vi "Parse ISO 8601 Timestring.vi"(8 "error in (no error)":errorcluster, 10 "ISO 8601 type":T1, 11 "ISO 8601 Timestring":string) -> (0 "error out":errorcluster, 3 "Time Stamp":timestamp)   [LabVIEW 2013]
uses:
  Controls/ISO 8601 Type.ctl
  Database.lvlib
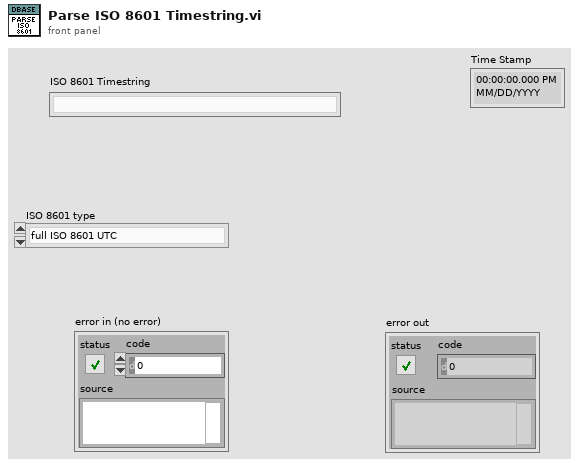
[diagram p1: front panel]
types:
  T1 = typedef "Database.lvlib/ISO 8601 Type.ctl" = enum16{"full ISO 8601 UTC", "Windows ISO 8601 UTC", "YYYY-MM-DD UTC"}
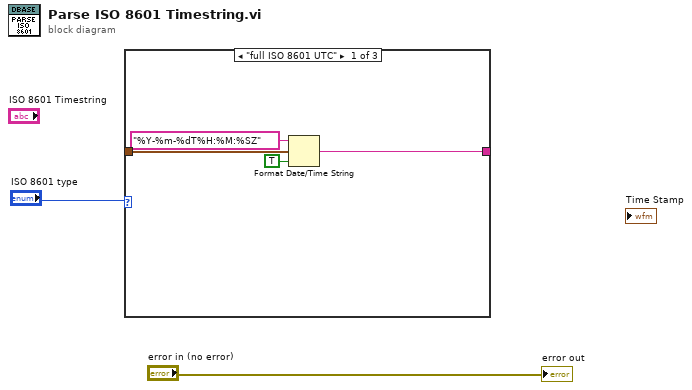
[diagram p0: block diagram]
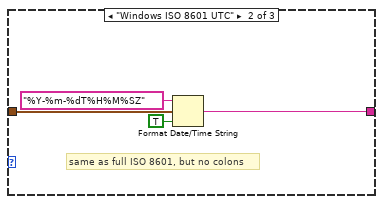
[diagram p2: hidden frame]
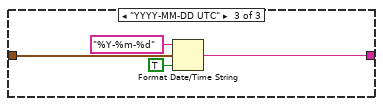
[diagram p3: hidden frame]
diagram:
  n1 = case shown="\"full ISO 8601 UTC\"" "ISO 8601 type" {
    tunnel: [w8 w12 w16] -> w3
    tunnel: [w6 w10 w14] -> w2
    frame "full ISO 8601 UTC" {
      n2 = Format Date/Time String(time format string (%c)="%Y-%m-%dT%H:%M:%SZ", seconds (now)=w8, UTC format=TRUE) -> (date/time string=w6:string)
    }
    frame "Windows ISO 8601 UTC" {
      # "same as full ISO 8601, but no colons"
      n3 = Format Date/Time String(time format string (%c)="%Y-%m-%dT%H%M%SZ", seconds (now)=w12, UTC format=TRUE) -> (date/time string=w10:string)
    }
    frame "YYYY-MM-DD UTC" {
      n4 = Format Date/Time String(time format string (%c)="%Y-%m-%d", seconds (now)=w16, UTC format=TRUE) -> (date/time string=w14:string)
    }
  }
  "error out" <- "error in (no error)"
